vi "BRig_RT__Case_Exp__State_CuePre__v4.vi"(0 "input_dataCurrent":u16[](array[numeric]), 1 "input_dataTrial":u16[][](array[numeric]), 3 "input_Cue2":bool, 6 "input_I_lick":bool, 9 "input_arrTrig":bool[](array[boolean])) -> (12 "output_state":T1, 13 "output_arrTrig":bool[](array[boolean]), 14 "output_dataCurrent":u16[](array[numeric]), 15 "output_dataTrial":u16[][](array[numeric]))   [LabVIEW 2014]
uses:
  myRIO_BRig_RT__Case_Exp_stateList.ctl
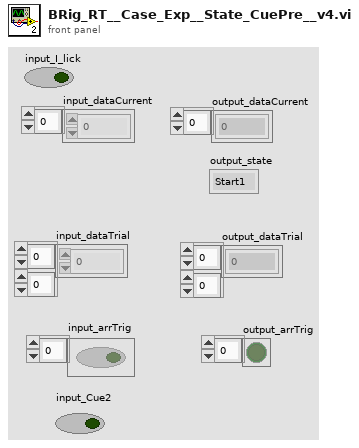
[diagram p1: front panel]
types:
  T1 = typedef "myRIO_BRig_RT__Case_Exp_stateList.ctl" = enum16{"Start1", "Start2", "Start3", "saveSettings1", "saveSettings2", "saveSettings3", "saveSettings4", "saveSettings_LC_ENL_l1", "saveSettings_LC_ENL_l2", "saveSettings_LC_Cue_l1", "saveSettings_LC_Cue_l2", "saveSettings6_LC_l1_Other", "SaveSettings6_LC_l2_Other", "setSettings_Audio", "setSettings_Laser", "initBlock_pre", "initBlock", "initBlock2", "initBlock_post", "initTrial_pre", "initTrial", "initTrial2", "initTrial3", "initTrial4", "initTrial_LC_ENL1", "initTrial_LC_Cue1", "initTrial_LC_Cue1_2", "initTrial_LC_Sel", "initTrial_post", "ENL1_pre", "ENL1", "ENL1_post", "ENL1Penalty_pre", "ENL1Penalty", "ENL2_pre", "ENL2", "ENL2Penalty_pre", "ENL2Penalty", "Cue1_pre", "Cue1", "Cue1_post", "Cue1Penalty_pre", "Cue1Penalty", "Cue2_pre", "Cue2", "Cue2Penalty_pre", "Cue2Penalty", "Selection_pre", "Selection", "Select_post", "SelectReward_pre", "SelectReward", "SelectRewardPost_pre", "SelectRewardPost", "SelectWrong_pre", "SelectWrong", "SelectWrong_post", "SelectTimeout_pre", "SelectTimeout", "SelectTimeout_post", "endTrial_pre", "endTrial1", "endTrial2", "endTrial3", "endTrial_post", "endBlock_pre", "endBlock", "endBlock_post", "endExp", "commConnect", "commUpload_pre", "commUpload_dataBlock", "commUpload_dataCurrent", "commUpload_dataExp", "commUpload_dataLC", "commUpload_dataTrial", "commUpload_post", "saveData_pre", "saveData_dataBlock", "saveData_dataCurrent", "saveData_dataExp", "saveData_dataLC", "saveData_dataTrial", "saveData_post", "empty_endBlock1", "empty_endBlock2", "empty_endTrial1", "empty_endTrial2", "empty_endTrial3", "empty_endTrial4", "empty_endTrial5", "dummyState", "dummyState_endBlock", "FreeReward_pre", "FreeReward", "FreeRewardPost_pre", "FreeRewardPost"}
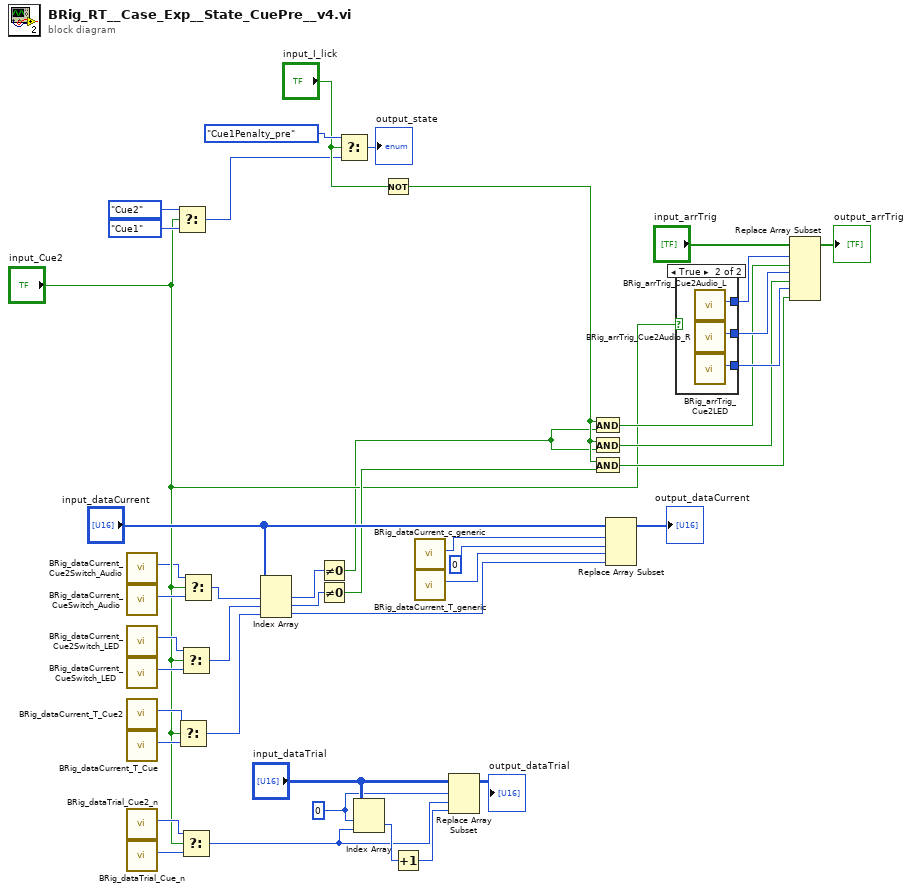
[diagram p0: block diagram]
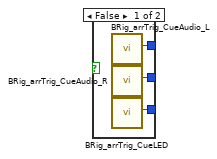
[diagram p2: hidden frame]
diagram:
  w18 = 0
  n1 = call "BRig_dataCurrent_Cue2Switch_Audio.vi"() -> ("output_Cue2Switch_Audio"=w3:i32)  [unwired: 11 in]
  n2 = call "BRig_dataCurrent_CueSwitch_Audio.vi"() -> ("output_CueSwitch_Audio"=w5:i32)  [unwired: 11 in]
  n3 = call "BRig_dataCurrent_Cue2Switch_LED.vi"() -> ("output_Cue2Switch_LED"=w8:i32)  [unwired: 11 in]
  n4 = call "BRig_dataCurrent_CueSwitch_LED.vi"() -> ("output_CueSwitch_LED"=w7:i32)  [unwired: 11 in]
  n5 = call "BRig_dataCurrent_T_Cue2.vi"() -> ("output_T_Cue2"=w13:i32)  [unwired: 11 in]
  n6 = call "BRig_dataCurrent_T_Cue.vi"() -> ("output_T_Cue"=w14:i32)  [unwired: 11 in]
  n7 = call "BRig_dataTrial_Cue2_n.vi"() -> ("output_Cue2_n"=w10:i32)  [unwired: 11 in]
  n8 = call "BRig_dataTrial_Cue_n.vi"() -> ("output_Cue_n"=w11:i32)  [unwired: 11 in]
  n9 = Select(t=myRIO_BRig_RT__Case_Exp_stateList."Cue2", s="input_Cue2", f=myRIO_BRig_RT__Case_Exp_stateList."Cue1" ("Enum")) -> (s? t:f=w16:T1)
  n10 = Select(t=w13, s="input_Cue2", f=w14) -> (s? t:f=w12:i32)
  n11 = Select(t=w8, s="input_Cue2", f=w7) -> (s? t:f=w6:i32)
  n12 = Select(t=w10, s="input_Cue2", f=w11) -> (s? t:f=w9:i32)
  n13 = Select(t=w3, s="input_Cue2", f=w5) -> (s? t:f=w2:i32)
  n14 = Index Array(array="input_dataCurrent", index #1=w2, index #2=w6, index #3=w12) -> (element #1=w35:u16, element #2=w34:u16, element #3=w36:u16)
  n15 = Not Equal To 0?(x=w35) -> (x != 0?=w1:bool)
  n16 = Not Equal To 0?(x=w34) -> (x != 0?=w32:bool)
  n17 = Select(t=myRIO_BRig_RT__Case_Exp_stateList."Cue1Penalty_pre" ("Enum"), s="input_I_lick", f=w16) -> (s? t:f=→"output_state":T1)
  n18 = Index Array(array="input_dataTrial", index (row)=w18, index (col)=w9) -> (element=w29:u16)
  n19 = Not(x="input_I_lick") -> (.not. x?=w31:bool)
  n20 = Increment(x=w29) -> (x+1=w28:u16)
  n21 = call "BRig_dataCurrent_c_generic.vi"() -> ("output_count_generic"=w39:i32)  [unwired: 11 in]
  n22 = call "BRig_dataCurrent_T_generic.vi"() -> ("output_T_generic"=w38:i32)  [unwired: 11 in]
  n23 = Replace Array Subset(array="input_dataTrial", new element=w28, index (row)=w18, index (col)=w9) -> (→"output_dataTrial":u16[][])
  n24 = And(x=w31, y=w1) -> (x .and. y?=w20:bool)
  n25 = And(x=w31, y=w1) -> (x .and. y?=w21:bool)
  n26 = And(x=w31, y=w32) -> (x .and. y?=w22:bool)
  n27 = Replace Array Subset(array="input_dataCurrent", new element #1=u16 0 ("new element/subarray"), index #1=w39, new element #2=w36, index #2=w38) -> (→"output_dataCurrent":u16[])
  n28 = case shown="True" "input_Cue2" {
    tunnel: [w46 w49] -> w25
    tunnel: [w45 w48] -> w24
    tunnel: [w44 w47] -> w23
    frame False {
      n29 = call "BRig_arrTrig_CueAudio_L.vi"() -> ("output_CueAudio_L"=w46:i32)  [unwired: 11 in]
      n30 = call "BRig_arrTrig_CueAudio_R.vi"() -> ("output_CueAudio_R"=w45:i32)  [unwired: 11 in]
      n31 = call "BRig_arrTrig_CueLED.vi"() -> ("output_CueLED"=w44:i32)  [unwired: 11 in]
    }
    frame True {
      n32 = call "BRig_arrTrig_Cue2Audio_L.vi"() -> ("output_Cue2Audio_L"=w49:i32)  [unwired: 11 in]
      n33 = call "BRig_arrTrig_Cue2Audio_R.vi"() -> ("output_Cue2Audio_R"=w48:i32)  [unwired: 11 in]
      n34 = call "BRig_arrTrig_Cue2LED.vi"() -> ("output_Cue2LED"=w47:i32)  [unwired: 11 in]
    }
  }
  n35 = Replace Array Subset(array="input_arrTrig", new element #1=w20, index #1=w25, new element #2=w21, index #2=w24, new element #3=w22, index #3=w23) -> (→"output_arrTrig":bool[])
